vi "Tree Test -3.vi"() -> ()   [LabVIEW 2015]
panel:
  in  "number":i32
  out "Single Selection Display Text":string
  in  "Single Selection Tree":string(tree)="Sine Graph"
  in  "Stop":bool
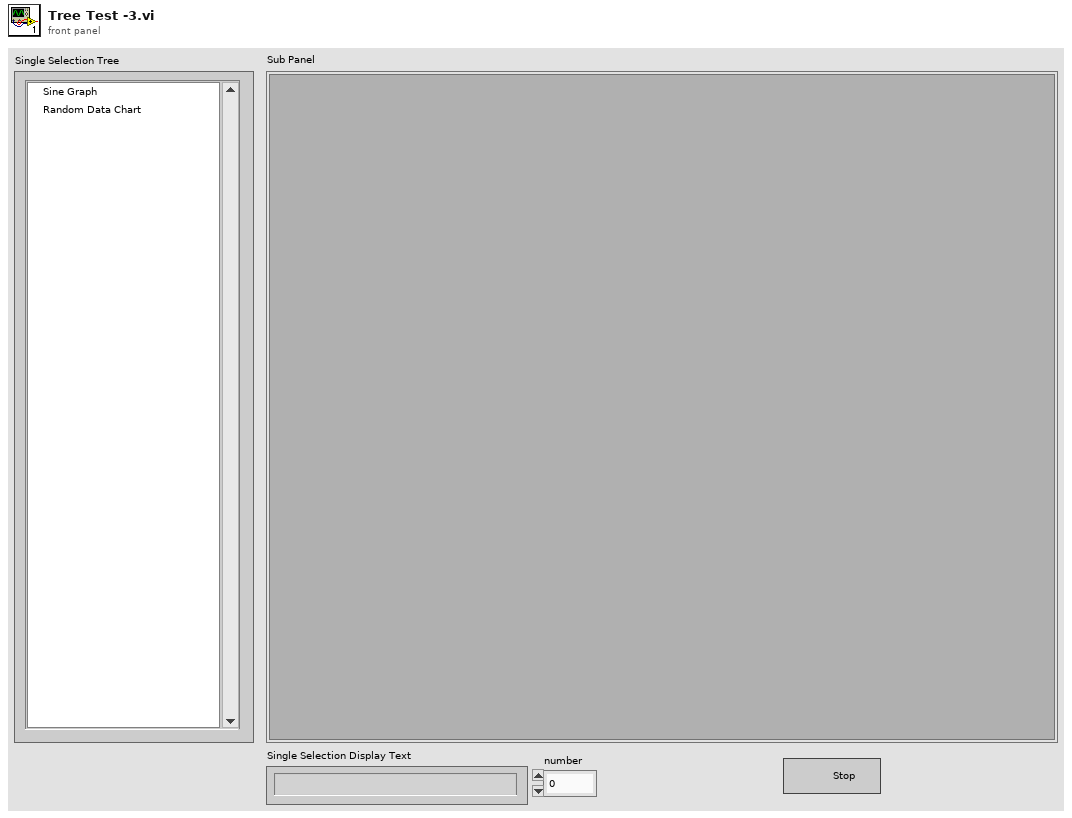
[diagram p1: front panel]
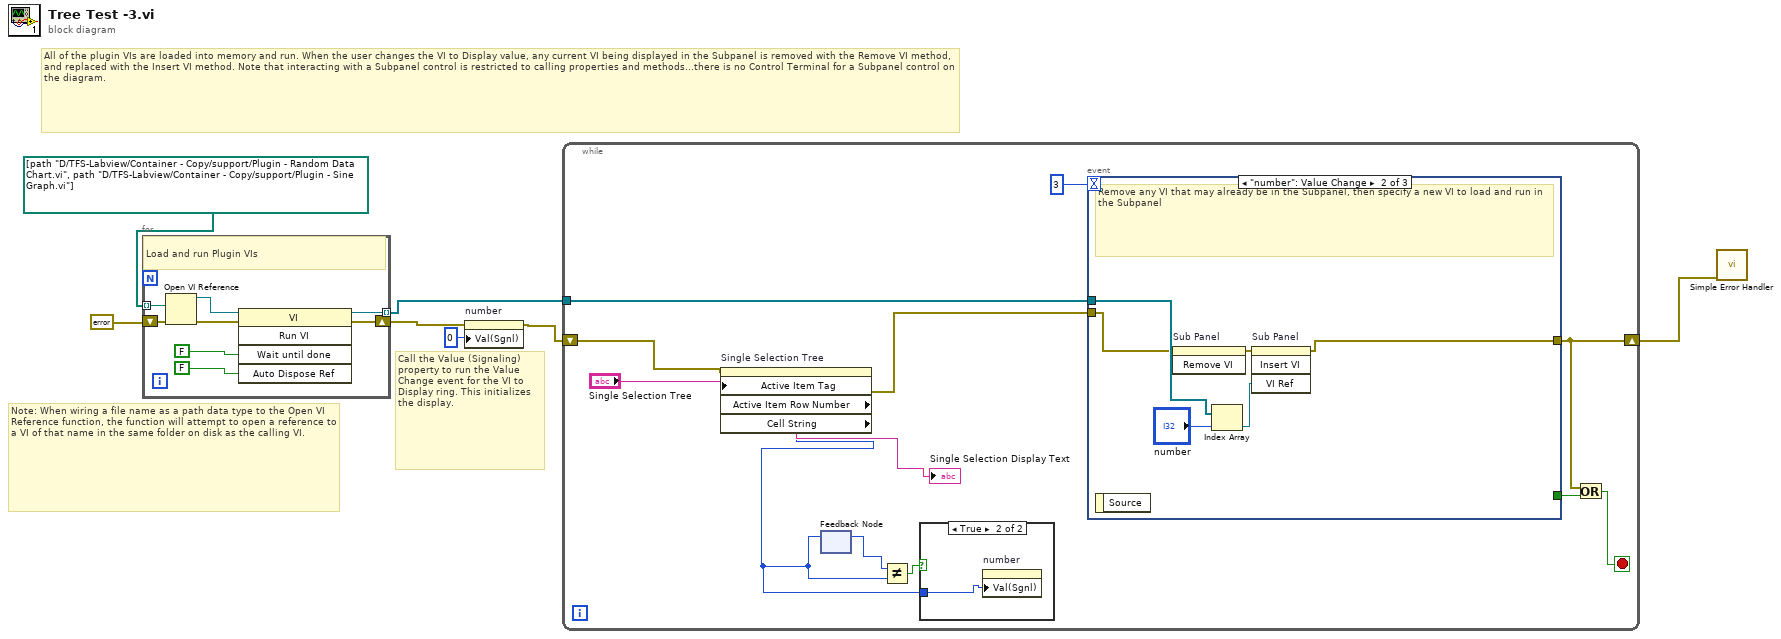
[diagram p0: block diagram]
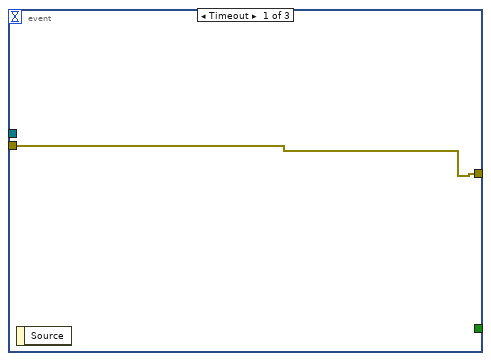
[diagram p3: hidden frame]
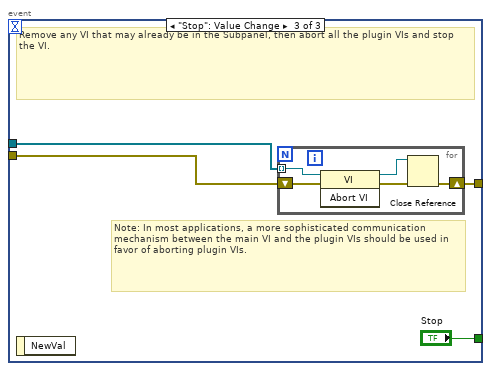
[diagram p4: hidden frame]
diagram:
  # "All of the plugin VIs are loaded into memory and run. When the user changes the VI to Display value, any current VI being displayed in the Subpanel is removed with the Remove VI method, and replaced with the Insert VI method. Note that interacting with a Subpanel control is restricted to calling properties and methods...there is no Control Terminal for a Subpanel control on the diagram."
  # "Note: When wiring a file name as a path data type to the Open VI Reference function, the function will attempt to open a reference to a VI of that name in the same folder on disk as the calling VI."
  # "Call the Value (Signaling) property to run the Value Change event for the VI to Display ring. This initializes the display."
  n1 = for {
    tunnel: path[] [path "D:/TFS-Labview/Container - Copy/support/Plugin - Random Data Chart.vi", path "D:/TFS-Labview/Container - Copy/support/Plugin - Sine Graph.vi"] -> [w11] mode=indexing
    tunnel: [w10] -> w6 mode=indexing
    shift-right: [w8] -> w3
    shift-left: errorcluster {"status"=FALSE, "code"=0, "source"=""} ("error constant") -> [w9]
    # "Load and run Plugin VIs"
    n2 = Open VI Reference(vi path=w11, error in (no error)=w9) -> (vi reference=w12:refnum<vi>, error out=w13:errorcluster)  [unwired: 4 in]
    n3 = invoke class="VI" method="Run VI"(reference=w12, error in=w13, "Wait until done"=FALSE ("Wait Until Done"), "Auto Dispose Ref"=FALSE ("Auto Dispose Reference")) -> (reference out=w10:refnum<vi>, error out=w8:errorcluster)  [unwired: 1 in, 3 out]
  }
  n4 = property on="number" class="DigNum (strict)"(error in=w3, "Val(Sgnl)"=0 ("Value (Signaling)")) -> (error out=w2:errorcluster)  [unwired: 1 in, 1 out]
  n5 = while {
    tunnel: w6 -> [w26]
    shift-right: [w27] -> w7
    shift-left: w2 -> [w25]
    stop <- w19 stop-if-true
    n6 = property on="Single Selection Tree" class="TreeControl (strict)"(error in=w25, "Active Item Tag"="Single Selection Tree") -> (error out=w21:errorcluster, "Active Item Row Number"=w16:i32, "Cell String"=→"Single Selection Display Text":string)  [unwired: 1 in, 1 out]
    n7 = feedback #1() -> (w18:i32)  [unwired: 1 in]
    n8 = feedback-in #1(w16) -> ()
    n9 = Not Equal?(x=w18, y=w16) -> (x != y?=w17:bool)
    n10 = case shown="True" w17 {
      tunnel: w16 -> [_ w28]
      frame False {
      }
      frame True {
        n11 = property on="number" class="DigNum (strict)"("Val(Sgnl)"=w28) -> ()  [unwired: 2 in, 2 out]
      }
    }
    n12 = event shown="[1] \"number\": Value Change" {
      selector: _ -> [_ _ _]
      dyn-events: _ -> [_ _ _]
      timeout: 3 -> [_ _ _]
      tunnel: [_ _ "Stop"] -> w20
      tunnel: [w29 w33 w37] -> w27
      tunnel: w26 -> [_ w35 w38]
      tunnel: w21 -> [w29 w31 w36]
      event Timeout {
        n13 = event-data() -> ()  [unwired: 1 in, 1 out]
      }
      event "number": Value Change {
        # "Remove any VI that may already be in the Subpanel, then specify a new VI to load and run in the Subpanel"
        n14 = event-data() -> ()  [unwired: 1 in, 1 out]
        n15 = invoke on="Sub Panel" class="SubPnl" method="Remove VI"(error in=w31) -> (error out=w32:errorcluster)  [unwired: 2 in, 2 out]
        n16 = Index Array(array=w35, index="number") -> (element=w34:refnum<vi>)
        n17 = invoke on="Sub Panel" class="SubPnl" method="Insert VI"(error in=w32, "VI Ref"=w34) -> (error out=w33:errorcluster)  [unwired: 2 in, 3 out]
      }
      event "Stop": Value Change {
        # "Note: In most applications, a more sophisticated communication mechanism between the main VI and the plugin VIs should be used in favor of aborting plugin VIs."
        # "Remove any VI that may already be in the Subpanel, then abort all the plugin VIs and stop the VI."
        n18 = event-data() -> ()  [unwired: 1 in, 1 out]
        n19 = for {
          shift-right: [w40] -> w37
          shift-left: w36 -> [w44]
          tunnel: w38 -> [w43] mode=indexing
          n20 = invoke class="VI" method="Abort VI"(reference=w43, error in=w44) -> (reference out=w41:refnum<vi>, error out=w42:errorcluster)  [unwired: 1 in, 1 out]
          n21 = Close Reference(reference=w41, error in (no error)=w42) -> (error out=w40:errorcluster)
        }
      }
    }
    n22 = Or(x=w27, y=w20) -> (x .or. y?=w19:bool)
  }
  n23 = call <vilib>:"Simple Error Handler.vi"("error in (no error)"=w7) -> ()  [unwired: 4 in, 5 out]
